vi "SV UFF58 Format ASCII Function Header.vi"(0 "record 11 - z-axis data characteristics":T2={"specific data type"=0, "length units exponent"=0, "force units exponent"=0, "temperature units exponent"=0, "axis label"="NONE", "axis units label"="NONE"} {"specific data type" items=["unknown"=0, "general"=1, "stress"=2, "strain"=3, "temperature"=5, "heat flux"=6, "displacement"=8, "reaction force"=9, "velocity"=11, "acceleration"=12, "excitation force"=13, "pressure"=15, "mass"=16, "time"=17, "frequency"=18, "rpm"=19, "order"=20, "sound pressure"=21, "sound intensity"=22, "sound power"=23]}, 4 "record 10 - ordinate denominator data characteristics":T2={"specific data type"=0, "length units exponent"=0, "force units exponent"=0, "temperature units exponent"=0, "axis label"="NONE", "axis units label"="NONE"} {"specific data type" items=["unknown"=0, "general"=1, "stress"=2, "strain"=3, "temperature"=5, "heat flux"=6, "displacement"=8, "reaction force"=9, "velocity"=11, "acceleration"=12, "excitation force"=13, "pressure"=15, "mass"=16, "time"=17, "frequency"=18, "rpm"=19, "order"=20, "sound pressure"=21, "sound intensity"=22, "sound power"=23]}, 6 "record 9 - ordinate data characteristics":T2={"specific data type"=0, "length units exponent"=0, "force units exponent"=0, "temperature units exponent"=0, "axis label"="NONE", "axis units label"="NONE"} {"specific data type" items=["unknown"=0, "general"=1, "stress"=2, "strain"=3, "temperature"=5, "heat flux"=6, "displacement"=8, "reaction force"=9, "velocity"=11, "acceleration"=12, "excitation force"=13, "pressure"=15, "mass"=16, "time"=17, "frequency"=18, "rpm"=19, "order"=20, "sound pressure"=21, "sound intensity"=22, "sound power"=23]}, 8 "record 8 - abscissa data characteristics":T2={"specific data type"=0, "length units exponent"=0, "force units exponent"=0, "temperature units exponent"=0, "axis label"="NONE", "axis units label"="NONE"} {"specific data type" items=["unknown"=0, "general"=1, "stress"=2, "strain"=3, "temperature"=5, "heat flux"=6, "displacement"=8, "reaction force"=9, "velocity"=11, "acceleration"=12, "excitation force"=13, "pressure"=15, "mass"=16, "time"=17, "frequency"=18, "rpm"=19, "order"=20, "sound pressure"=21, "sound intensity"=22, "sound power"=23]}, 9 "record 7 - data form":T7={"ordinate data type"=4, "number of data values/pairs"=0, "abscissa spacing"=enum."even", "abscissa minimum"=0.0, "abscissa increment"=1.0, "z-axis value"=0.0} {"ordinate data type" items=["real single precision"=2, "real double precision"=4, "complex single precision"=5, "complex double precision"=6]}, 10 "record 6 - DOF identification":T4={"function type"=enum."time response", "function ID number"=0, "version number"=0, "load case ID number"=0, "response entity name"="NONE", "response node"=0, "response direction"=0, "reference entity name"="NONE", "reference node"=0, "reference direction"=0} {"reference direction" items=["-Z Rotation"=-6, "-Y Rotation"=-5, "-X Rotation"=-4, "-Z Translation"=-3, "-Y Translation"=-2, "-X Translation"=-1, "Scalar"=0, "+X Translation"=1, "+Y Translation"=2, "+Z Translation"=3, "+X Rotation"=4, "+Y Rotation"=5, "+Z Rotation"=6]; "response direction" items=["-Z Rotation"=-6, "-Y Rotation"=-5, "-X Rotation"=-4, "-Z Translation"=-3, "-Y Translation"=-2, "-X Translation"=-1, "Scalar"=0, "+X Translation"=1, "+Y Translation"=2, "+Z Translation"=3, "+X Rotation"=4, "+Y Rotation"=5, "+Z Rotation"=6]}, 11 "records (1-5)":T1={"ID line 1"="NONE", "ID line 2"="NONE", "ID line 3 (date & time)"="NONE", "ID line 4"="NONE", "ID line 5"="NONE"}) -> (3 "formatted UFF58 ASCII header":string)   [LabVIEW 2017, in "SoundVib_UFF58.lvlib"]
doc: "Formats records 1-11 to the UFF58 (universal file format) ASCII header format. Wire the <B>formatted UFF58 ASCII header</B> output to the <B>formatted UFF58 ASCII header</B> input of the SV UFF58 Format ASCII Ordinate Data (Evenly Spaced) VI. You also can use this VI in combination with Read VIs found in UFF58b Advanced VIs to convert a function header from a binary UFF58 file to an ASCII function header."
uses:
  <vilib>/addons/Sound and Vibration/svt_UFF58/SoundVib_UFF58.lvlib
  <vilib>/addons/Sound and Vibration/svt_UFF58/subVIs/sv_UFF58 Axis Characteristics.ctl
  <vilib>/addons/Sound and Vibration/svt_UFF58/subVIs/sv_UFF58 Specific Datatype.ctl
  <vilib>/addons/Sound and Vibration/svt_UFF58/subVIs/sv_UFF58 DOF.ctl
  <vilib>/addons/Sound and Vibration/svt_UFF58/subVIs/sv_FunctionType.ctl
  <vilib>/addons/Sound and Vibration/svt_UFF58/subVIs/sv_UFF58 Response Direction.ctl
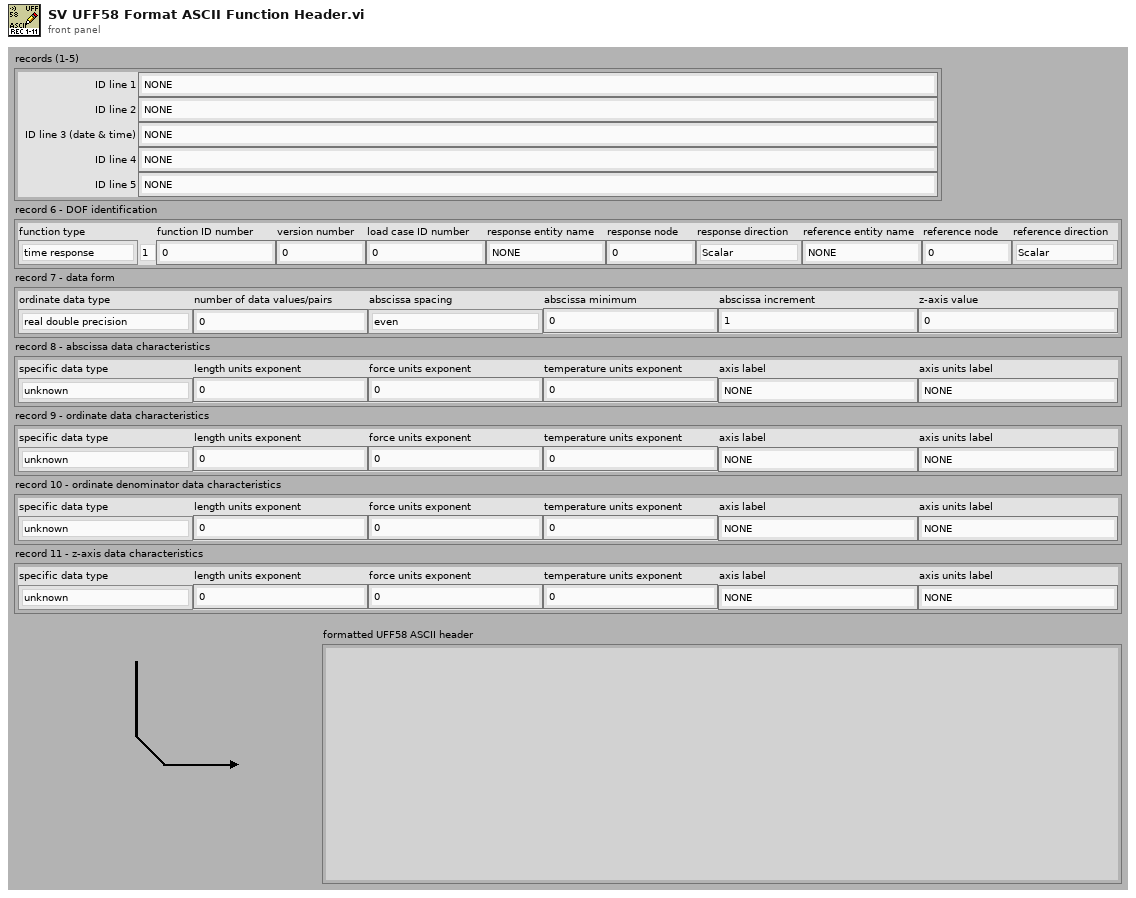
[diagram p1: front panel]
types:
  T1 = cluster{"ID line 1":string, "ID line 2":string, "ID line 3 (date & time)":string, "ID line 4":string, "ID line 5":string}
  T2 = typedef "SoundVib_UFF58.lvlib/sv_UFF58 Axis Characteristics.ctl" = cluster{"specific data type":T3, "length units exponent":i32, "force units exponent":i32, "temperature units exponent":i32, "axis label":string, "axis units label":string}
  T3 = typedef "SoundVib_UFF58.lvlib/sv_UFF58 Specific Datatype.ctl" = u16
  T4 = typedef "SoundVib_UFF58.lvlib/sv_UFF58 DOF.ctl" = cluster{"function type":T5, "function ID number":i32, "version number":i32, "load case ID number":i32, "response entity name":string, "response node":i32, "response direction":T6, "reference entity name":string, "reference node":i32, "reference direction":T6}
  T5 = typedef "SoundVib_UFF58.lvlib/sv_FunctionType.ctl" = enum16{"general or unknown", "time response", "auto spectrum", "cross spectrum", "frequency response function", "transmissibility", "coherence", "auto correlation", "cross correlation", "power spectral density (PSD)", "energy spectral density (ESD)", "probability density function", "spectrum", "cumulative frequency distribution", "peaks valley", "stress/cycles", "strain/cycles", "orbit", "mode indicator function", "force pattern", "partial power", "partial coherence", "eigenvalue", "eigenvector", "shock response spectrum", "finite impulse response filter", "multiple coherence", "order function", "phase compensation"}
  T6 = typedef "SoundVib_UFF58.lvlib/sv_UFF58 Response Direction.ctl" = i32
  T7 = cluster{"ordinate data type":u16, "number of data values/pairs":i32, "abscissa spacing":enum16{"uneven", "even"}, "abscissa minimum":dbl, "abscissa increment":dbl, "z-axis value":dbl}
  T8 = cluster{"ID line 1":bool, "ID line 2":bool, "ID line 3 (date & time)":bool, "ID line 4":bool, "ID line 5":bool}
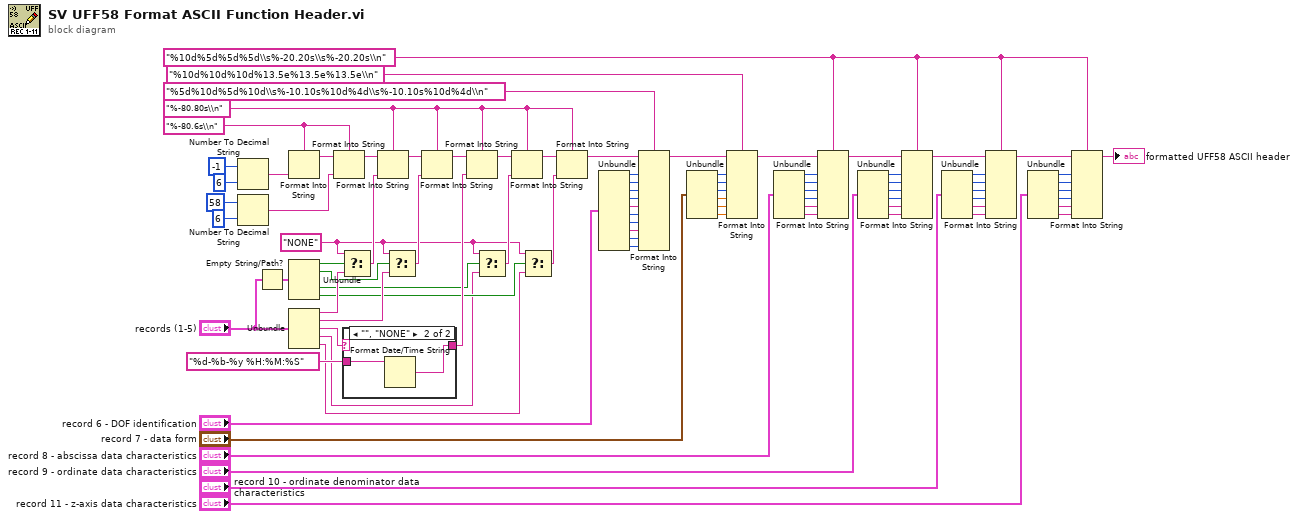
[diagram p0: block diagram]
diagram:
  w1 = "NONE" ("format string")
  w82 = "%-80.6s\\n" ("format string")
  w79 = "%10d%5d%5d%5d\\s%-20.20s\\s%-20.20s\\n" ("format string")
  w78 = "%-80.80s\\n" ("format string")
  n1 = Number To Decimal String(number=-1, width (-)=i16 6) -> (decimal integer string=w83:string)
  n2 = Number To Decimal String(number=58, width (-)=i16 6) -> (decimal integer string=w84:string)
  n3 = Empty String/Path?(string/path="records (1-5)") -> (empty?=w18:T8)
  n4 = Format Into String(format string=w82, w83) -> (resulting string=w35:string)  [unwired: 2 in, 1 out]
  n5 = Unbundle(w18) -> ("ID line 1"=w17:bool, "ID line 2"=w4:bool, "ID line 4"=w12:bool, "ID line 5"=w7:bool)  [unwired: 1 out]
  n6 = Unbundle("records (1-5)") -> ("ID line 1"=w16:string, "ID line 2"=w14:string, "ID line 3 (date & time)"=w20:string, "ID line 4"=w3:string, "ID line 5"=w6:string)
  n7 = Format Into String(format string=w82, initial string=w35, w84) -> (resulting string=w34:string)  [unwired: 1 in, 1 out]
  n8 = Select(t=w1, s=w17, f=w16) -> (s? t:f=w15:string)
  n9 = case shown="\"\", \"NONE\"" w20 {
    selector: w20 -> [w89 _]
    tunnel: "%d-%b-%y %H:%M:%S" ("time format string (%c)") -> [_ w91]
    tunnel: [w89 w90] -> w21
    frame Default {
    }
    frame "", "NONE" {
      n10 = Format Date/Time String(time format string (%c)=w91) -> (date/time string=w90:string)  [unwired: 2 in]
    }
  }
  n11 = Format Into String(format string=w78, initial string=w34, w15) -> (resulting string=w33:string)  [unwired: 1 in, 1 out]
  n12 = Select(t=w1, s=w4, f=w14) -> (s? t:f=w13:string)
  n13 = Format Into String(format string=w78, initial string=w33, w13) -> (resulting string=w32:string)  [unwired: 1 in, 1 out]
  n14 = Format Into String(format string=w78, initial string=w32, w21) -> (resulting string=w31:string)  [unwired: 1 in, 1 out]
  n15 = Select(t=w1, s=w12, f=w3) -> (s? t:f=w2:string)
  n16 = Format Into String(format string=w78, initial string=w31, w2) -> (resulting string=w30:string)  [unwired: 1 in, 1 out]
  n17 = Select(t=w1, s=w7, f=w6) -> (s? t:f=w5:string)
  n18 = Format Into String(format string=w78, initial string=w30, w5) -> (resulting string=w29:string)  [unwired: 1 in, 1 out]
  n19 = Unbundle("record 6 - DOF identification") -> ("function type"=w46:T5, "function ID number"=w47:i32, "version number"=w48:i32, "load case ID number"=w49:i32, "response entity name"=w50:string, "response node"=w51:i32, "response direction"=w11:T6, "reference entity name"=w10:string, "reference node"=w9:i32, "reference direction"=w8:T6)
  n20 = Format Into String(format string="%5d%10d%5d%10d\\s%-10.10s%10d%4d\\s%-10.10s%10d%4d\\n", initial string=w29, w46, w47, w48, w49, w50, w51, w11, w10, w9, w8) -> (resulting string=w28:string)  [unwired: 1 in, 1 out]
  n21 = Unbundle("record 7 - data form") -> ("ordinate data type"=w44:u16, "number of data values/pairs"=w53:i32, "abscissa spacing"=w54:enum16{"uneven", "even"}, "abscissa minimum"=w55:dbl, "abscissa increment"=w56:dbl, "z-axis value"=w36:dbl)
  n22 = Format Into String(format string="%10d%10d%10d%13.5e%13.5e%13.5e\\n", initial string=w28, w44, w53, w54, w55, w56, w36) -> (resulting string=w27:string)  [unwired: 1 in, 1 out]
  n23 = Unbundle("record 8 - abscissa data characteristics") -> ("specific data type"=w59:T3, "length units exponent"=w58:i32, "force units exponent"=w60:i32, "temperature units exponent"=w61:i32, "axis label"=w62:string, "axis units label"=w63:string)
  n24 = Format Into String(format string=w79, initial string=w27, w59, w58, w60, w61, w62, w63) -> (resulting string=w26:string)  [unwired: 1 in, 1 out]
  n25 = Unbundle("record 9 - ordinate data characteristics") -> ("specific data type"=w68:T3, "length units exponent"=w69:i32, "force units exponent"=w67:i32, "temperature units exponent"=w66:i32, "axis label"=w65:string, "axis units label"=w64:string)
  n26 = Format Into String(format string=w79, initial string=w26, w68, w69, w67, w66, w65, w64) -> (resulting string=w25:string)  [unwired: 1 in, 1 out]
  n27 = Unbundle("record 10 - ordinate denominator data characteristics") -> ("specific data type"=w70:T3, "length units exponent"=w77:i32, "force units exponent"=w71:i32, "temperature units exponent"=w72:i32, "axis label"=w73:string, "axis units label"=w74:string)
  n28 = Format Into String(format string=w79, initial string=w25, w70, w77, w71, w72, w73, w74) -> (resulting string=w24:string)  [unwired: 1 in, 1 out]
  n29 = Unbundle("record 11 - z-axis data characteristics") -> ("specific data type"=w43:T3, "length units exponent"=w42:i32, "force units exponent"=w41:i32, "temperature units exponent"=w40:i32, "axis label"=w39:string, "axis units label"=w38:string)
  n30 = Format Into String(format string=w79, initial string=w24, w43, w42, w41, w40, w39, w38) -> (resulting string=→"formatted UFF58 ASCII header":string)  [unwired: 1 in, 1 out]
